vi "Format Address.vi"(10 "Address":T1) -> (2 "Formatted Address":string)   [LabVIEW 2020, in "Gmail API.lvlib" / "Gmail.lvclass"]
uses:
  Gmail.lvclass
  Mail Address.ctl
  Gmail.lvclass/Gmail.ctl
  Gmail API.lvlib
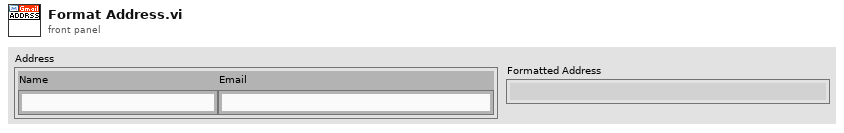
[diagram p1: front panel]
types:
  T1 = typedef "Gmail API.lvlib/Mail Address.ctl" = cluster{"Name":string, "Email":string}
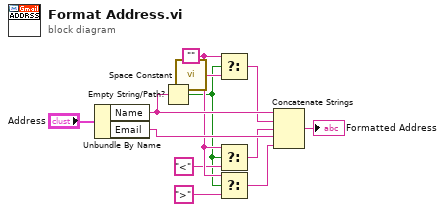
[diagram p0: block diagram]
diagram:
  w4 = ""
  n1 = Unbundle By Name("Address") -> ("Name"=w11:string, "Email"=w9:string)
  n2 = Empty String/Path?(string/path=w11) -> (empty?=w1:bool)
  n3 = call <vilib>:"Space Constant.vi"() -> ("String"=w12:string)
  n4 = Select(t=w4, s=w1, f=w12) -> (s? t:f=w10:string)
  n5 = Select(t=w4, s=w1, f="<") -> (s? t:f=w6:string)
  n6 = Select(t=w4, s=w1, f=">") -> (s? t:f=w5:string)
  n7 = Concatenate Strings(w11, w10, w6, w9, w5) -> (→"Formatted Address":string)
